vi "Main Tclk.vi"() -> ()   [LabVIEW 2018] (continued)
        n4080 = Select(t=u32[] [16448250, 16711422, 16645629, 16579836, 16514043, 16448250, 16382457, 16316664, 16250871, 16185078, 16119285, 16053492, 15987699, 15921906, 15856113, 15790320, 15724527, 15658734, 15592941, 15527148, 15461355, 15395562, 15329769, 15263976, 15198183, 15132390, 15066597, 15000804, 14935011, 14869218, 14803425, 14737632, 14671839, 14606046, 14540253, 14474460, 14408667, 14342874, 14277081, 14211288, 14145495, 14079702, 14013909, 13948116, 13882323, 13816530, 13750737, 13684944, 13619151, 13553358, 13487565, 13421772, 13355979, 13290186, 13224393, 13158600, 13092807, 13027014, 12961221, 12895428, 12829635, 12763842, 12698049, 12632256, 12566463, 12500670, 12434877, 12369084, 12303291, 12237498, 12171705, 12105912, 12040119, 11974326, 11908533, 11842740, 11776947, 11711154, 11645361, 11579568, 11513775, 11447982, 11382189, 11316396, 11250603, 11184810, 11119017, 11053224, 10987431, 10921638, 10855845, 10790052, 10724259, 10658466, 10592673, 10526880, 10461087, 10395294, 10329501, 10263708, 10197915, 10132122, 10066329, 10000536, 9934743, 9868950, 9803157, 9737364, 9671571, 9605778, 9539985, 9474192, 9408399, 9342606, 9276813, 9211020, 9145227, 9079434, 9013641, 8947848, 8882055, 8816262, 8750469, 8684676, 8618883, 8553090, 8487297, 8421504, 8355711, 8289918, 8224125, 8158332, 8092539, 8026746, 7960953, 7895160, 7829367, 7763574, 7697781, 7631988, 7566195, 7500402, 7434609, 7368816, 7303023, 7237230, 7171437, 7105644, 7039851, 6974058, 6908265, 6842472, 6776679, 6710886, 6645093, 6579300, 6513507, 6447714, 6381921, 6316128, 6250335, 6184542, 6118749, 6052956, 5987163, 5921370, 5855577, 5789784, 5723991, 5658198, 5592405, 5526612, 5460819, 5395026, 5329233, 5263440, 5197647, 5131854, 5066061, 5000268, 4934475, 4868682, 4802889, 4737096, 4671303, 4605510, 4539717, 4473924, 4408131, 4342338, 4276545, 4210752, 4144959, 4079166, 4013373, 3947580, 3881787, 3815994, 3750201, 3684408, 3618615, 3552822, 3487029, 3421236, 3355443, 3289650, 3223857, 3158064, 3092271, 3026478, 2960685, 2894892, 2829099, 2763306, 2697513, 2631720, 2565927, 2500134, 2434341, 2368548, 2302755, 2236962, 2171169, 2105376, 2039583, 1973790, 1907997, 1842204, 1776411, 1710618, 1644825, 1579032, 1513239, 1447446, 1381653, 1315860, 1250067, 1184274, 1118481, 1052688, 986895, 921102, 855309, 789516, 723723, 657930, 592137, 526344, 460551, 394758, 328965, 263172, 197379, 131586, 65793, 16777222] ("256 gray scale inverse"), s=w2804, f=u32[] [16777222, 65793, 131586, 197379, 263172, 328965, 394758, 460551, 526344, 592137, 657930, 723723, 789516, 855309, 921102, 986895, 1052688, 1118481, 1184274, 1250067, 1315860, 1381653, 1447446, 1513239, 1579032, 1644825, 1710618, 1776411, 1842204, 1907997, 1973790, 2039583, 2105376, 2171169, 2236962, 2302755, 2368548, 2434341, 2500134, 2565927, 2631720, 2697513, 2763306, 2829099, 2894892, 2960685, 3026478, 3092271, 3158064, 3223857, 3289650, 3355443, 3421236, 3487029, 3552822, 3618615, 3684408, 3750201, 3815994, 3881787, 3947580, 4013373, 4079166, 4144959, 4210752, 4276545, 4342338, 4408131, 4473924, 4539717, 4605510, 4671303, 4737096, 4802889, 4868682, 4934475, 5000268, 5066061, 5131854, 5197647, 5263440, 5329233, 5395026, 5460819, 5526612, 5592405, 5658198, 5723991, 5789784, 5855577, 5921370, 5987163, 6052956, 6118749, 6184542, 6250335, 6316128, 6381921, 6447714, 6513507, 6579300, 6645093, 6710886, 6776679, 6842472, 6908265, 6974058, 7039851, 7105644, 7171437, 7237230, 7303023, 7368816, 7434609, 7500402, 7566195, 7631988, 7697781, 7763574, 7829367, 7895160, 7960953, 8026746, 8092539, 8158332, 8224125, 8289918, 8355711, 8421504, 8487297, 8553090, 8618883, 8684676, 8750469, 8816262, 8882055, 8947848, 9013641, 9079434, 9145227, 9211020, 9276813, 9342606, 9408399, 9474192, 9539985, 9605778, 9671571, 9737364, 9803157, 9868950, 9934743, 10000536, 10066329, 10132122, 10197915, 10263708, 10329501, 10395294, 10461087, 10526880, 10592673, 10658466, 10724259, 10790052, 10855845, 10921638, 10987431, 11053224, 11119017, 11184810, 11250603, 11316396, 11382189, 11447982, 11513775, 11579568, 11645361, 11711154, 11776947, 11842740, 11908533, 11974326, 12040119, 12105912, 12171705, 12237498, 12303291, 12369084, 12434877, 12500670, 12566463, 12632256, 12698049, 12763842, 12829635, 12895428, 12961221, 13027014, 13092807, 13158600, 13224393, 13290186, 13355979, 13421772, 13487565, 13553358, 13619151, 13684944, 13750737, 13816530, 13882323, 13948116, 14013909, 14079702, 14145495, 14211288, 14277081, 14342874, 14408667, 14474460, 14540253, 14606046, 14671839, 14737632, 14803425, 14869218, 14935011, 15000804, 15066597, 15132390, 15198183, 15263976, 15329769, 15395562, 15461355, 15527148, 15592941, 15658734, 15724527, 15790320, 15856113, 15921906, 15987699, 16053492, 16119285, 16185078, 16250871, 16316664, 16382457, 16448250, 16514043, 16579836, 16645629, 16711422, 16448250] ("256 gray scale")) -> (s? t:f=w2805:u32[])
        n4081 = property on="DetB e- Scaling" class="DigNum (strict)"("Visible"=w2652) -> ()  [unwired: 2 in, 2 out]
        n4082 = property on="Detector B" class="IntGraph (strict)"("Color Table"=w2805, "Caption.Text"=w2840) -> ()  [unwired: 2 in, 2 out]
        n4083 = property on="Det A" class="IntGraph (strict)"("Color Table"=w2806) -> ()  [unwired: 2 in, 2 out]
        n4084 = property on="Align failed array" class="Arr (strict)"("Index Values"=w2701) -> ()  [unwired: 2 in, 2 out]
        n4085 = property on="WD (mm)" class="Arr (strict)"("Index Values"=w2701) -> ()  [unwired: 2 in, 2 out]
        n4086 = property on="X stig" class="Arr (strict)"("Index Values"=w2701) -> ()  [unwired: 2 in, 2 out]
        n4087 = property on="Y stig" class="Arr (strict)"("Index Values"=w2701) -> ()  [unwired: 2 in, 2 out]
        n4088 = property on="X aln" class="Arr (strict)"("Index Values"=w2701) -> ()  [unwired: 2 in, 2 out]
        n4089 = property on="Y aln" class="Arr (strict)"("Index Values"=w2701) -> ()  [unwired: 2 in, 2 out]
        n4090 = property on="Det B" class="IntGraph (strict)"("Color Table"=w2805) -> ()  [unwired: 2 in, 2 out]
        n4091 = property on="Detector A Low Mag" class="IntGraph (strict)"("Color Table"=w2806) -> ()  [unwired: 2 in, 2 out]
        n4092 = local read "FIB"() -> (w2654:bool)
        n4093 = local read "Mill"() -> (w2653:bool)
        n4094 = property on="Detector B Low Mag" class="IntGraph (strict)"("Color Table"=w2805) -> ()  [unwired: 2 in, 2 out]
        n4095 = Or(x=w2654, y=w2653) -> (x .or. y?=w2655:bool)
        n4096 = shared-variable ".\\Zeiss Library.lvlib\\Milling Z Voltage RT"() -> (w2733:sgl)  [unwired: 1 in, 1 out]
        "Milling Z realtime (V)" <- w2733
        n4097 = case shown="True" w2655 {
          tunnel: w2733 -> [_ w2953]
          frame False {
          }
          frame True {
            n4098 = control-ref of="FIB Image"() -> (w2957:refnum<vi>)
            n4099 = local read "FIB Scan Parameters"() -> (w2955:T32)
            n4100 = local read "FIB Options"() -> (w2954:T33)
            n4101 = local read "Milling para"() -> (w2956:T35)
            n4102 = call "FIB image draw milling.vi"("Milling Z Voltage"=w2953, "Milling para"=w2956, "FIB Options"=w2954, "FIB Scan Parameters"=w2955, "Image reference"=w2957) -> ()  [unwired: 5 in, 2 out]
          }
        }
        n4103 = property on="Det A LM" class="IntGraph (strict)"("Color Table"=w2806) -> ()  [unwired: 2 in, 2 out]
        n4104 = property on="Det B LM" class="IntGraph (strict)"("Color Table"=w2805) -> ()  [unwired: 2 in, 2 out]
      }
      n4105 = Open VI Reference(vi path=w709) -> (vi reference=w714:refnum<vi>, error out=w708:errorcluster)  [unwired: 1 in, 4 out]
      n4106 = register-events(error in=w708, refnum<vi> refnum) -> (reference out=w711:refnum<event-registration>)  [unwired: 1 in, 1 out]
      n4107 = local read "Trapezoidal"() -> (w706:cluster{"X":i16, "Y":i16}[])
      n4108 = while {
        stop <- w718 stop-if-true
        n4109 = Wait Until Next ms Multiple(millisecond multiple=u32 100) -> ()  [unwired: 1 out]
        n4110 = case shown="True" "Scan x1" {
          frame False {
          }
          frame True {
            n4111 = Two Button Dialog(message="Single SEM Scan?") -> (T button?=w719:bool)  [unwired: 2 in]
            n4112 = case shown="True" w719 {
              frame False {
                n4113 = local write "Scan x1"(FALSE ("Scan")) -> ()
              }
              frame True {
                n4114 = stacked-sequence {
                  frame #0 {
                    n4115 = local read "SEM Scan Parameters"() -> (w727:T26)
                    n4116 = Unbundle By Name(w727) -> ("WD (mm)"=w728:sgl[][], "X stig"=w731:sgl[][], "Y stig"=w734:sgl[][], "X aln"=w735:sgl[][], "Y aln"=w737:sgl[][], "dX (um)"=w739:sgl[], "dY (um)"=w742:sgl[], "Y tiles"=w724:u8, "X tiles"=w723:u8)
                    n4117 = local read "WD Stig Aln tile offsets"() -> (w725:T3)
                    n4118 = Array Size(array=w728) -> (size(s)=w729:i32[])
                    n4119 = Array Size(array=w731) -> (size(s)=w730:i32[])
                    n4120 = Array Size(array=w734) -> (size(s)=w733:i32[])
                    n4121 = Array Size(array=w735) -> (size(s)=w732:i32[])
                    n4122 = Array Size(array=w737) -> (size(s)=w736:i32[])
                    n4123 = Array Size(array=w739) -> (size(s)=w740:i32)
                    n4124 = Array Size(array=w742) -> (size(s)=w741:i32)
                    n4125 = Build Array(w724, w723) -> (w738:u8[])
                    n4126 = Equal?(x=w729, y=w738) -> (x = y?=w743:bool[])
                    n4127 = Equal?(x=w730, y=w738) -> (x = y?=w744:bool[])
                    n4128 = Equal?(x=w733, y=w738) -> (x = y?=w746:bool[])
                    n4129 = Equal?(x=w732, y=w738) -> (x = y?=w747:bool[])
                    n4130 = Equal?(x=w736, y=w738) -> (x = y?=w748:bool[])
                    n4131 = Equal?(x=w740, y=w724) -> (x = y?=w749:bool)
                    n4132 = Equal?(x=w741, y=w723) -> (x = y?=w750:bool)
                    n4133 = Build Array (concatenate)(w743, w744, w746, w747, w748, w749, w750) -> (w745:bool[])
                    n4134 = And Array Elements(Boolean array=w745) -> (logical AND=w722:bool)
                    n4135 = case shown="True" w722 {
                      tunnel: [w751 w779] -> w726
                      tunnel: w727 -> [w753 w773]
                      tunnel: w725 -> [w752 w760]
                      frame False {
                        w755 = sgl 0.0 ("element")
                        n4136 = Unbundle By Name(w753) -> ("Y tiles"=w757:u8, "X tiles"=w759:u8)
                        n4137 = Initialize Array(w755, w757, w759) -> (w758:sgl[][])
                        n4138 = Initialize Array(w755, w757) -> (w756:sgl[])
                        n4139 = Initialize Array(w755, w759) -> (w754:sgl[])
                        n4140 = Bundle By Name(cluster=w752, "dWD"=w758, "dX stig"=w758, "dY stig"=w758, "dX aln"=w758, "dY aln"=w758, "dX (um)"=w756, "dY (um)"=w754) -> (w751:T3)
                      }
                      frame True {
                        n4141 = Unbundle By Name(w773) -> ("WD (mm)"=w769:sgl[][], "X stig"=w767:sgl[][], "Y stig"=w764:sgl[][], "X aln"=w763:sgl[][], "Y aln"=w761:sgl[][], "dX (um)"=w780:sgl[], "dY (um)"=w785:sgl[], "Y tiles"=w772:u8, "X tiles"=w771:u8)
                        n4142 = expression code="(x-1)/2"(w772) -> (w783:u8)
                        n4143 = expression code="(x-1)/2"(w771) -> (w786:u8)
                        n4144 = Index Array(array=w769, index (row)=w783, index (col)=w786) -> (element=w770:sgl)
                        n4145 = Index Array(array=w767, index (row)=w783, index (col)=w786) -> (element=w768:sgl)
                        n4146 = Index Array(array=w764, index (row)=w783, index (col)=w786) -> (element=w765:sgl)
                        n4147 = Index Array(array=w763, index (row)=w783, index (col)=w786) -> (element=w766:sgl)
                        n4148 = Index Array(array=w761, index (row)=w783, index (col)=w786) -> (element=w762:sgl)
                        n4149 = Index Array(array=w780, index=w783) -> (element=w781:sgl)
                        n4150 = Index Array(array=w785, index=w786) -> (element=w784:sgl)
                        n4151 = Subtract(x=w769, y=w770) -> (x-y=w774:sgl[][])
                        n4152 = Subtract(x=w767, y=w768) -> (x-y=w775:sgl[][])
                        n4153 = Subtract(x=w764, y=w765) -> (x-y=w776:sgl[][])
                        n4154 = Subtract(x=w763, y=w766) -> (x-y=w777:sgl[][])
                        n4155 = Subtract(x=w761, y=w762) -> (x-y=w778:sgl[][])
                        n4156 = Subtract(x=w780, y=w781) -> (x-y=w782:sgl[])
                        n4157 = Subtract(x=w785, y=w784) -> (x-y=w787:sgl[])
                        n4158 = Bundle By Name(cluster=w760, "dWD"=w774, "dX stig"=w775, "dY stig"=w776, "dX aln"=w777, "dY aln"=w778, "dX (um)"=w782, "dY (um)"=w787) -> (w779:T3)
                      }
                    }
                    n4159 = local write "WD Stig Aln tile offsets"(w726) -> ()
                  }
                  frame #1 {
                    n4160 = local read "SEM Scan Parameters"() -> (w793:T26)
                    n4161 = Unbundle By Name(w793) -> ("X tiles"=w789:u8, "Y tiles"=w790:u8)
                    n4162 = Multiply(x=w789, y=w790) -> (x*y=w791:u8)
                    n4163 = Greater?(x=w791, y=u8 1) -> (0:w792:bool)
                    n4164 = case shown="True" w792 {
                      frame False {
                      }
                      frame True {
                        n4165 = local read "Api"() -> (w811:refnum<k7>)
                        n4166 = call "SmartSEM Remote API get float.vi"("lpszParam"="AP_WD", "ActiveX Container"=w811) -> ("error out"=w822:errorcluster, "vValue"=w809:sgl)  [unwired: 7 in, 1 out]
                        n4167 = call "SmartSEM Remote API get float.vi"("error in"=w822, "lpszParam"="AP_STIG_X", "ActiveX Container"=w811) -> ("error out"=w823:errorcluster, "vValue"=w816:sgl, "reference out"=w813:refnum<k7>)  [unwired: 6 in]
                        n4168 = local read "WD Stig Aln tile offsets"() -> (w806:T3)
                        n4169 = expression code="x*1000"(w809) -> (w807:sgl)
                        n4170 = Unbundle By Name(w806) -> ("dWD"=w805:sgl[][], "dX stig"=w804:sgl[][], "dY stig"=w803:sgl[][], "dX aln"=w802:sgl[][], "dY aln"=w801:sgl[][])
                        n4171 = call "SmartSEM Remote API get float.vi"("error in"=w823, "lpszParam"="AP_APERTURE_ALIGN_X", "ActiveX Container"=w813) -> ("error out"=w824:errorcluster, "vValue"=w815:sgl)  [unwired: 6 in, 1 out]
                        n4172 = call "SmartSEM Remote API get float.vi"("error in"=w824, "lpszParam"="AP_STIG_Y", "ActiveX Container"=w811) -> ("error out"=w818:errorcluster, "vValue"=w821:sgl, "reference out"=w817:refnum<k7>)  [unwired: 6 in]
                        n4173 = call "SmartSEM Remote API get float.vi"("error in"=w818, "lpszParam"="AP_APERTURE_ALIGN_Y", "ActiveX Container"=w817) -> ("vValue"=w820:sgl)  [unwired: 6 in, 2 out]
                        n4174 = local read "SEM Scan Parameters"() -> (w799:T26)
                        n4175 = Add(x=w805, y=w807) -> (x+y=w798:sgl[][])
                        n4176 = Add(x=w804, y=w816) -> (x+y=w797:sgl[][])
                        n4177 = Add(x=w803, y=w821) -> (x+y=w796:sgl[][])
                        n4178 = Add(x=w802, y=w815) -> (x+y=w795:sgl[][])
                        n4179 = Add(x=w801, y=w820) -> (x+y=w794:sgl[][])
                        n4180 = Bundle By Name(cluster=w799, "WD (mm)"=w798, "X stig"=w797, "Y stig"=w796, "X aln"=w795, "Y aln"=w794) -> (w800:T26)
                        n4181 = local write "SEM Scan Parameters"(w800) -> ()
                      }
                    }
                  }
                  frame #2 {
                    n4182 = local read "SEM HW Config"() -> (w850:T9)
                    n4183 = local read "Detector Information"() -> (w849:T8)
                    n4184 = local read "SEM Scan Parameters"() -> (w837:T26)
                    n4185 = local read "SEM Options"() -> (w847:T27)
                    n4186 = local read "Focus Index Options"() -> (w846:T28)
                    n4187 = local read "File Information"() -> (w845:T31)
                    n4188 = local read "Milling para"() -> (w844:T35)
                    n4189 = Bundle By Name(cluster="Tiled scan inputs", "HW Config"=w850, "Det Info"=w849, "SEM Scan Parameters"=w837, "SEM Options"=w847, "Focus Index Options"=w846, "File Information"=w845, "Milling para"=w844, "Additional Info"=cluster{"Restart flag":u8, "Stage move flag":u8} {"Restart flag"=100, "Stage move flag"=100}) -> (w839:T6)
                    n4190 = Unbundle By Name(w837) -> ("X tiles"=w836:u8, "Y tiles"=w835:u8)
                    n4191 = Multiply(x=w836, y=w835) -> (x*y=w834:u8)
                    n4192 = Greater?(x=w834, y=u8 1) -> (0:w833:bool)
                    n4193 = local read "WatchDog Mode"() -> (w852:u16)
                    n4194 = case shown="True" w833 {
                      tunnel: w839 -> [w862 w865]
                      tunnel: [w862 w863] -> w838
                      frame False {
                      }
                      frame True {
                        w864 = TRUE ("SEM Options.Set WD")
                        n4195 = Bundle By Name(cluster=w865, "SEM Options.Set WD"=w864, "SEM Options.Set stig"=w864, "SEM Options.Set aln"=w864) -> (w863:T6)
                      }
                    }
                    n4196 = local read "Api"() -> (w851:refnum<k7>)
                    n4197 = call "2D scan tiled.vi"("WatchDog Mode"=w852, "Tiled scan inputs"=w838, "ActiveX Container"=w851) -> ("Image Focus Index Tiled"=w840:T53, "Image Focus Index Array Tiled"=w841:T54, "Single scan outputs"=w860:T55, "8-bit over scale"=w857:bool[])  [unwired: 3 in, 2 out]
                    n4198 = local read "FI Detector"() -> (w843:u16)
                    n4199 = Index Array(array=w857, index #1=0 ("index"), index #2=1 ("index")) -> (element #1=→"Det A over scale":bool, element #2=→"Det B over scale":bool)
                    n4200 = case shown="1" w843 {
                      tunnel: w840 -> [w869 w873 w877 w881]
                      tunnel: [w868 w870 w876 w880] -> w827
                      tunnel: w841 -> [w866 w872 w875 w879]
                      tunnel: [w867 w871 w874 w878] -> w842
                      frame 0, Default {
                        n4201 = Unbundle By Name(w869) -> ("A Img Focus Index"=w868:sgl[][])
                        n4202 = Unbundle By Name(w866) -> ("A Img Focus Index array"=w867:sgl[][][][])
                      }
                      frame 1 {
                        n4203 = Unbundle By Name(w873) -> ("B Img Focus Index"=w870:sgl[][])
                        n4204 = Unbundle By Name(w872) -> ("B Img Focus Index array"=w871:sgl[][][][])
                      }
                      frame 2 {
                        n4205 = Unbundle By Name(w877) -> ("C Img Focus Index"=w876:sgl[][])
                        n4206 = Unbundle By Name(w875) -> ("C Img Focus Index array"=w874:sgl[][][][])
                      }
                      frame 3 {
                        n4207 = Unbundle By Name(w881) -> ("D Img Focus Index"=w880:sgl[][])
                        n4208 = Unbundle By Name(w879) -> ("D Img Focus Index array"=w878:sgl[][][][])
                      }
                    }
                    n4209 = Unbundle By Name(w860) -> ("SEM Parameters"=→"SEM Parameters":T13, "Image Focus Index"=→"Image Focus Index":T14)
                    n4210 = Array Size(array=w827) -> (size(s)=w828:i32[])
                    n4211 = local write "Focus Index tiled"(w827) -> ()
                    n4212 = local write "Focus Index array tiled"(w842) -> ()
                    n4213 = local write "FRC resolution"(sgl 0.0 ("FRC resolution")) -> ()
                    n4214 = Multiply Array Elements(1:w828) -> (0:w829:i32)
                    n4215 = Reshape Array(w827, w829) -> (w830:sgl[])
                    n4216 = call-poly <vilib>:"Mean.vi"("X"=w830) -> ("mean"=w831:dbl)  [unwired: 1 out]
                    n4217 = local write "Focus Index"(w831) -> ()
                    "Status message" <- "SEM scanning" ("Status message")
                  }
                  frame #3 {
                    n4218 = local write "Scan x1"(FALSE ("Scan")) -> ()
                    n4219 = local write "Status message"("Single scan finished." ("Status message")) -> ()
                  }
                }
              }
            }
          }
        }
        n4220 = local read "Stop"() -> (w718:bool)
      }
      n4221 = while {
        tunnel: w711 -> [w3157]
        tunnel: [w3156] -> w712
        tunnel: [w3154] -> w713
        tunnel: w714 -> [w3155]
        shift-right: [w3149] -> _
        shift-left: w706 -> [w3148]
        stop <- w3153 stop-if-true
        n4222 = Wait Until Next ms Multiple(millisecond multiple=u32 1) -> ()  [unwired: 1 out]
        n4223 = event shown="[24] \"Mill\": Value Change" {
          selector: w3157 -> [_ _ _ _ _ _ _ _ _ _ _ _ _ _ _ _ _ _ _ _ _ _ _ _ _ _ _ _ _ _ _ _ w3973 _ w4176 _ _ _ _ _ _ _ _ _ _ _ _ _ _ _ _ _ _ _ _ _ _ _ _ _ _ _ _ _ _ _ _ _ _ _ _ _ _ _ _ _ _ _ _ _ _ _ _ _ _ _ _ _ _ _ _ _ _ _]
          dyn-events: [_ _ _ _ _ _ _ _ _ _ _ _ _ _ _ _ _ _ _ _ _ _ _ _ _ _ _ _ _ _ _ _ w3972 _ w4175 _ _ _ _ _ _ _ _ _ _ _ _ _ _ _ _ _ _ _ _ _ _ _ _ _ _ _ _ _ _ _ _ _ _ _ _ _ _ _ _ _ _ _ _ _ _ _ _ _ _ _ _ _ _ _ _ _ _ _] -> w3156
          timeout: _ -> [_ _ _ _ _ _ _ _ _ _ _ _ _ _ _ _ _ _ _ _ _ _ _ _ _ _ _ _ _ _ _ _ _ _ _ _ _ _ _ _ _ _ _ _ _ _ _ _ _ _ _ _ _ _ _ _ _ _ _ _ _ _ _ _ _ _ _ _ _ _ _ _ _ _ _ _ _ _ _ _ _ _ _ _ _ _ _ _ _ _ _ _ _ _]
          tunnel: [_ _ _ _ _ _ _ _ _ _ _ _ _ _ _ _ _ _ _ _ _ _ _ _ _ _ _ _ _ _ _ _ w3971 _ w4174 _ _ _ _ _ _ _ _ _ _ _ _ _ _ _ _ _ _ _ _ _ _ _ _ _ _ _ _ _ _ _ _ _ _ _ _ _ _ _ _ _ _ _ _ _ _ _ _ _ _ _ _ _ _ _ _ _ _ _] -> w3154
          tunnel: w3155 -> [_ _ _ _ _ _ _ _ _ _ _ _ _ _ _ _ _ _ _ _ _ _ _ _ _ _ _ _ _ _ _ _ w3969 _ _ _ _ _ _ _ _ _ _ _ _ _ _ _ _ _ _ _ _ _ _ _ _ _ _ _ _ _ _ _ _ _ _ _ _ _ _ _ _ _ _ _ _ _ _ _ _ _ _ _ _ _ _ _ _ _ _ _ _ _]
          tunnel: [_ _ _ _ _ _ _ _ _ _ _ w3510 _ _ _ _ _ _ _ _ _ _ _ _ _ _ _ _ _ _ _ _ _ _ _ _ _ _ _ _ _ _ _ _ _ _ _ _ _ _ _ _ _ _ _ _ _ _ _ _ _ _ _ _ _ _ _ _ _ _ _ _ _ _ _ _ _ _ _ _ _ _ _ _ _ _ _ _ _ _ _ _ _ _] -> w3151
          tunnel: [_ _ _ _ _ _ _ _ _ _ _ _ _ _ _ _ _ _ _ _ _ _ _ _ _ _ _ _ _ _ _ _ w3965 w3984 w4140 _ _ _ w4309 _ _ _ _ _ _ _ _ w4788 _ _ _ _ _ _ _ _ _ _ _ _ _ _ _ _ _ _ _ _ _ _ _ _ _ _ _ _ _ _ _ _ _ _ _ _ _ _ _ _ _ _ _ _ _ _] -> w3149
          tunnel: w3148 -> [_ _ _ _ _ _ _ _ _ _ _ _ _ _ _ _ _ _ _ _ _ _ _ _ _ _ _ _ _ _ _ _ w3965 w3983 w4140 _ _ _ _ _ _ _ _ _ _ _ _ w4787 _ _ _ _ _ _ _ _ _ _ _ _ _ _ _ _ _ _ _ _ _ _ _ _ _ _ _ _ _ _ _ _ _ _ _ _ _ _ _ _ _ _ _ _ _ _]
          event Timeout {
            n4224 = event-data() -> ()  [unwired: 3 out]
          }
          event Key Down? {
            # "Ignore Ctrl-W, Alt-F4"
            n4225 = event-data() -> ("Char"=w3169:i16, "VKey"=w3166:T48, "PlatMods"=w3164:T77)  [unwired: 7 out]
            n4226 = Unbundle By Name(w3164) -> ("Ctrl"=w3163:bool, "Alt"=w3161:bool)
            n4227 = Equal?(x=w3169, y=i16 119) -> (x = y?=w3167:bool)
            n4228 = Equal?(x=w3166, y=eventvkey."F4" ("VKey")) -> (x = y?=w3162:bool)
            n4229 = And(x=w3167, y=w3163) -> (x .and. y?=w3160:bool)
            n4230 = And(x=w3161, y=w3162) -> (x .and. y?=w3159:bool)
            n4231 = Compound Arithmetic op=OR(w3160, w3159) -> (w3158:bool)
            n4232 = event-data("Discard?"=w3158) -> ()  [unwired: 6 in, 1 out]
          }
          event "Hardware Configuration", "SEM Options", "Mid Mag SEM", "SEM Scan Parameters.Scan rate (Hz)", "SEM Scan Parameters.Oversampling", "SEM Scan Parameters.Oversampling auto", "SEM Scan Parameters.X size (um)", "SEM Scan Parameters.X size (V)", "SEM Scan Parameters.X size auto", "SEM Scan Parameters.Y size (um)", "SEM Scan Parameters.X center (um)", "SEM Scan Parameters.Y center (um)": Value Change {
            n4233 = event-data() -> ()  [unwired: 6 out]
            n4234 = local read "Hardware Configuration"() -> (w3178:T25)
            n4235 = local read "SEM Scan Parameters"() -> (w3194:T26)
            n4236 = local read "SEM Options"() -> (w3177:T27)
            n4237 = local read "SEM Status"() -> (w3176:T12)
            n4238 = local read "X full scale (V)"() -> (w3175:sgl)
            n4239 = local read "Mid Mag SEM"() -> (w3179:T29)
            n4240 = local read "SEM Mid Mag Scan Parameters"() -> (w3180:T5)
            n4241 = Unbundle By Name(w3179) -> ("X size (um)"=w3183:sgl, "Y size (um)"=w3184:sgl, "X center (um)"=w3185:dbl, "Y center (um)"=w3186:dbl, "Mid mag scan rate (Hz)"=w3181:u32, "Pixel size (nm)"=w3182:sgl)
            n4242 = call "SEM Scan Parameter Coerce.vi"("X full scale (V)"=w3175, "AI upper limit"=50000000.0, "SEM Status"=w3176, "SEM Options"=w3177, "SEM Scan Parameters"=w3194, "Hardware Configuration"=w3178) -> ("Coerced SEM Scan Parameters"=w3174:T5, "SEM FOV"=→"SEM FOV":dbl, "Detector number"=→"Detector number":i16)  [unwired: 3 in]
            n4243 = Bundle By Name(cluster=w3180, "X size (um)"=w3183, "Y size (um)"=w3184, "X center (um)"=w3185, "Y center (um)"=w3186, "Scan rate (Hz)"=w3181, "Pixel size (nm)"=w3182, "X size auto"=TRUE) -> (w3187:T5)
            n4244 = call "SEM Scan Parameter Coerce.vi"("X full scale (V)"=w3175, "SEM Status"=w3176, "SEM Options"=w3177, "SEM Scan Parameters"=w3187, "Hardware Configuration"=w3178) -> ("Coerced SEM Scan Parameters"=w3173:T5)  [unwired: 4 in, 2 out]
            n4245 = Unbundle By Name(w3173) -> ("X size (um)"=w3188:sgl, "Y size (um)"=w3189:sgl, "X center (um)"=w3190:dbl, "Y center (um)"=w3191:dbl, "Scan rate (Hz)"=w3192:u32, "Pixel size (nm)"=w3193:sgl)
            n4246 = Bundle By Name(cluster=w3179, "X size (um)"=w3188, "Y size (um)"=w3189, "X center (um)"=w3190, "Y center (um)"=w3191, "Mid mag scan rate (Hz)"=w3192, "Pixel size (nm)"=w3193) -> (w3172:T29)
            n4247 = local write "SEM Scan Parameters"(w3174) -> ()
            n4248 = local write "SEM Mid Mag Scan Parameters"(w3173) -> ()
            n4249 = local write "Mid Mag SEM"(w3172) -> ()
          }
          event "Scan x1": Value Change {
            n4250 = event-data() -> ()  [unwired: 6 out]
          }
          event "3D FIB-SEM": Value Change {
            n4251 = event-data() -> ("NewVal"=w3197:bool)  [unwired: 5 out]
            n4252 = case shown="False" w3197 {
              frame False {
                n4253 = Two Button Dialog(message="Stop 3D FIB-SEM?") -> (T button?=w3198:bool)  [unwired: 2 in]
                n4254 = local write "Mill Stop"(w3198) -> ()
                n4255 = case shown="True" w3198 {
                  frame False {
                    n4256 = local write "3D FIB-SEM"(TRUE ("3D FIB-SEM")) -> ()
                  }
                  frame True {
                    n4257 = stacked-sequence {
                      frame #0 {
                        n4258 = shared-variable "My Computer\\Zeiss Library.lvlib\\Milling Stop"(TRUE ("Milling Stop")) -> ()  [unwired: 1 in, 1 out]
                        n4259 = Wait (ms)(milliseconds to wait=u32 1000) -> ()  [unwired: 1 out]
                        n4260 = local write "Status message"("3D FIB-SEM stopped" ("Status message")) -> ()
                        n4261 = local read "WatchDog Mode"() -> (w3201:u16)
                        n4262 = call "FM Gen Pulse for FIB-SEM.vi"("WatchDog Mode"=w3201, "State Value"=i16 7) -> ()  [unwired: 7 in, 3 out]
                      }
                      frame #1 {
                        w3206 = FALSE ("3D FIB-SEM")
                        n4263 = local read "Last FIB recipe"() -> (w3216:path)
                        n4264 = local read "Email recipents file"() -> (w3210:path)
                        n4265 = local read "FIB Image"() -> (w3221:i16[][])
                        n4266 = Array Size(array=w3221) -> (size(s)=w3220:i32[])
                        n4267 = local write "Pause for reheat"(w3206) -> ()
                        n4268 = local write "3D FIB-SEM"(w3206) -> ()
                        n4269 = local write "FIB"(w3206) -> ()
                        n4270 = Add Array Elements(numeric array=w3220) -> (sum=w3219:i32)
                        n4271 = Not Equal To 0?(x=w3219) -> (x != 0?=w3218:bool)
                        n4272 = Open/Create/Replace File(file path (use dialog)=w3216) -> (error out=w3214:errorcluster)  [unwired: 5 in, 2 out]
                        n4273 = case shown="True" w3218 {
                          tunnel: w3221 -> [_ w3247]
                          frame False {
                          }
                          frame True {
                            n4274 = local read "Last FIB image"() -> (w3250:path)
                            n4275 = call "16bit Image Normalization.vi"("Transpose"=FALSE, "Input image"=w3247) -> ("Normalized image"=w3246:u8[][])  [unwired: 5 in, 4 out]
                            n4276 = call <vilib>:"Flatten Pixmap.vi"("colors"=u32[] [16777222, 65793, 131586, 197379, 263172, 328965, 394758, 460551, 526344, 592137, 657930, 723723, 789516, 855309, 921102, 986895, 1052688, 1118481, 1184274, 1250067, 1315860, 1381653, 1447446, 1513239, 1579032, 1644825, 1710618, 1776411, 1842204, 1907997, 1973790, 2039583, 2105376, 2171169, 2236962, 2302755, 2368548, 2434341, 2500134, 2565927, 2631720, 2697513, 2763306, 2829099, 2894892, 2960685, 3026478, 3092271, 3158064, 3223857, 3289650, 3355443, 3421236, 3487029, 3552822, 3618615, 3684408, 3750201, 3815994, 3881787, 3947580, 4013373, 4079166, 4144959, 4210752, 4276545, 4342338, 4408131, 4473924, 4539717, 4605510, 4671303, 4737096, 4802889, 4868682, 4934475, 5000268, 5066061, 5131854, 5197647, 5263440, 5329233, 5395026, 5460819, 5526612, 5592405, 5658198, 5723991, 5789784, 5855577, 5921370, 5987163, 6052956, 6118749, 6184542, 6250335, 6316128, 6381921, 6447714, 6513507, 6579300, 6645093, 6710886, 6776679, 6842472, 6908265, 6974058, 7039851, 7105644, 7171437, 7237230, 7303023, 7368816, 7434609, 7500402, 7566195, 7631988, 7697781, 7763574, 7829367, 7895160, 7960953, 8026746, 8092539, 8158332, 8224125, 8289918, 8355711, 8421504, 8487297, 8553090, 8618883, 8684676, 8750469, 8816262, 8882055, 8947848, 9013641, 9079434, 9145227, 9211020, 9276813, 9342606, 9408399, 9474192, 9539985, 9605778, 9671571, 9737364, 9803157, 9868950, 9934743, 10000536, 10066329, 10132122, 10197915, 10263708, 10329501, 10395294, 10461087, 10526880, 10592673, 10658466, 10724259, 10790052, 10855845, 10921638, 10987431, 11053224, 11119017, 11184810, 11250603, 11316396, 11382189, 11447982, 11513775, 11579568, 11645361, 11711154, 11776947, 11842740, 11908533, 11974326, 12040119, 12105912, 12171705, 12237498, 12303291, 12369084, 12434877, 12500670, 12566463, 12632256, 12698049, 12763842, 12829635, 12895428, 12961221, 13027014, 13092807, 13158600, 13224393, 13290186, 13355979, 13421772, 13487565, 13553358, 13619151, 13684944, 13750737, 13816530, 13882323, 13948116, 14013909, 14079702, 14145495, 14211288, 14277081, 14342874, 14408667, 14474460, 14540253, 14606046, 14671839, 14737632, 14803425, 14869218, 14935011, 15000804, 15066597, 15132390, 15198183, 15263976, 15329769, 15395562, 15461355, 15527148, 15592941, 15658734, 15724527, 15790320, 15856113, 15921906, 15987699, 16053492, 16119285, 16185078, 16250871, 16316664, 16382457, 16448250, 16514043, 16579836, 16645629, 16711422, 16448250] ("256 gray scale"), "8-bit pixmap"=w3246) -> ("image data"=w3249:T52)  [unwired: 4 in, 5 out]
                            n4277 = call <vilib>:"Write PNG File.vi"("image data"=w3249, "path to PNG file"=w3250) -> ()  [unwired: 1 in, 9 out]
                          }
                        }
                        n4278 = File/Directory Info(path=w3210) -> (path out=w3207:path, error out=w3209:errorcluster)  [unwired: 1 in, 5 out]
                        n4279 = Unbundle By Name(w3214) -> ("status"=w3215:bool)
                        n4280 = Unbundle By Name(w3209) -> ("status"=w3208:bool)
                        n4281 = local read "Recipe input"() -> (w3212:T7)
                        n4282 = case shown="False" w3215 {
                          tunnel: w3216 -> [w3244 w3245]
                          tunnel: [w3243 w3245] -> w3213
                          frame False {
                            n4283 = Delete(path (use dialog)=w3244) -> (deleted path=w3243:path)  [unwired: 4 in, 2 out]
                          }
                          frame True {
                          }
                        }
                        n4284 = case shown="False" w3208 {
                          tunnel: w3207 -> [w3230 _]
                          frame False {
                            n4285 = Delete(path (use dialog)=w3230) -> ()  [unwired: 4 in, 3 out]
                          }
                          frame True {
                          }
                        }
                        n4286 = call "Recipe read write.vi"("Write"=TRUE, "Recipe path"=w3213, "Write input"=w3212) -> ()  [unwired: 5 in, 4 out]
                        n4287 = local read "Detector A Low Mag"() -> (w3223:i16[][])
                        n4288 = local read "Detector B Low Mag"() -> (w3222:i16[][])
                        n4289 = Array Size(array=w3223) -> (size(s)=w3224:i32[])
                        n4290 = Array Size(array=w3222) -> (size(s)=w3229:i32[])
                        n4291 = Add Array Elements(numeric array=w3224) -> (sum=w3225:i32)
                        n4292 = Add Array Elements(numeric array=w3229) -> (sum=w3228:i32)
                        n4293 = Not Equal To 0?(x=w3225) -> (x != 0?=w3226:bool)
                        n4294 = Not Equal To 0?(x=w3228) -> (x != 0?=w3227:bool)
                        n4295 = case shown="True" w3226 {
                          tunnel: w3223 -> [_ w3239]
                          frame False {
                          }
                          frame True {
                            n4296 = local read "Last Det A Low Mag"() -> (w3241:path)
                            n4297 = call "16bit Image Normalization.vi"("Transpose"=FALSE, "Input image"=w3239) -> ("Normalized image"=w3238:u8[][])  [unwired: 5 in, 4 out]
                            n4298 = call <vilib>:"Flatten Pixmap.vi"("colors"=u32[] [16777222, 65793, 131586, 197379, 263172, 328965, 394758, 460551, 526344, 592137, 657930, 723723, 789516, 855309, 921102, 986895, 1052688, 1118481, 1184274, 1250067, 1315860, 1381653, 1447446, 1513239, 1579032, 1644825, 1710618, 1776411, 1842204, 1907997, 1973790, 2039583, 2105376, 2171169, 2236962, 2302755, 2368548, 2434341, 2500134, 2565927, 2631720, 2697513, 2763306, 2829099, 2894892, 2960685, 3026478, 3092271, 3158064, 3223857, 3289650, 3355443, 3421236, 3487029, 3552822, 3618615, 3684408, 3750201, 3815994, 3881787, 3947580, 4013373, 4079166, 4144959, 4210752, 4276545, 4342338, 4408131, 4473924, 4539717, 4605510, 4671303, 4737096, 4802889, 4868682, 4934475, 5000268, 5066061, 5131854, 5197647, 5263440, 5329233, 5395026, 5460819, 5526612, 5592405, 5658198, 5723991, 5789784, 5855577, 5921370, 5987163, 6052956, 6118749, 6184542, 6250335, 6316128, 6381921, 6447714, 6513507, 6579300, 6645093, 6710886, 6776679, 6842472, 6908265, 6974058, 7039851, 7105644, 7171437, 7237230, 7303023, 7368816, 7434609, 7500402, 7566195, 7631988, 7697781, 7763574, 7829367, 7895160, 7960953, 8026746, 8092539, 8158332, 8224125, 8289918, 8355711, 8421504, 8487297, 8553090, 8618883, 8684676, 8750469, 8816262, 8882055, 8947848, 9013641, 9079434, 9145227, 9211020, 9276813, 9342606, 9408399, 9474192, 9539985, 9605778, 9671571, 9737364, 9803157, 9868950, 9934743, 10000536, 10066329, 10132122, 10197915, 10263708, 10329501, 10395294, 10461087, 10526880, 10592673, 10658466, 10724259, 10790052, 10855845, 10921638, 10987431, 11053224, 11119017, 11184810, 11250603, 11316396, 11382189, 11447982, 11513775, 11579568, 11645361, 11711154, 11776947, 11842740, 11908533, 11974326, 12040119, 12105912, 12171705, 12237498, 12303291, 12369084, 12434877, 12500670, 12566463, 12632256, 12698049, 12763842, 12829635, 12895428, 12961221, 13027014, 13092807, 13158600, 13224393, 13290186, 13355979, 13421772, 13487565, 13553358, 13619151, 13684944, 13750737, 13816530, 13882323, 13948116, 14013909, 14079702, 14145495, 14211288, 14277081, 14342874, 14408667, 14474460, 14540253, 14606046, 14671839, 14737632, 14803425, 14869218, 14935011, 15000804, 15066597, 15132390, 15198183, 15263976, 15329769, 15395562, 15461355, 15527148, 15592941, 15658734, 15724527, 15790320, 15856113, 15921906, 15987699, 16053492, 16119285, 16185078, 16250871, 16316664, 16382457, 16448250, 16514043, 16579836, 16645629, 16711422, 16448250] ("256 gray scale"), "8-bit pixmap"=w3238) -> ("image data"=w3240:T52)  [unwired: 4 in, 5 out]
                            n4299 = call <vilib>:"Write PNG File.vi"("image data"=w3240, "path to PNG file"=w3241) -> ()  [unwired: 1 in, 9 out]
                          }
                        }
                        n4300 = case shown="True" w3227 {
                          tunnel: w3222 -> [_ w3232]
                          frame False {
                          }
                          frame True {
                            n4301 = local read "Last Det B Low Mag"() -> (w3235:path)
                            n4302 = call "16bit Image Normalization.vi"("Transpose"=FALSE, "Input image"=w3232) -> ("Normalized image"=w3231:u8[][])  [unwired: 5 in, 4 out]
                            n4303 = call <vilib>:"Flatten Pixmap.vi"("colors"=u32[] [16777222, 65793, 131586, 197379, 263172, 328965, 394758, 460551, 526344, 592137, 657930, 723723, 789516, 855309, 921102, 986895, 1052688, 1118481, 1184274, 1250067, 1315860, 1381653, 1447446, 1513239, 1579032, 1644825, 1710618, 1776411, 1842204, 1907997, 1973790, 2039583, 2105376, 2171169, 2236962, 2302755, 2368548, 2434341, 2500134, 2565927, 2631720, 2697513, 2763306, 2829099, 2894892, 2960685, 3026478, 3092271, 3158064, 3223857, 3289650, 3355443, 3421236, 3487029, 3552822, 3618615, 3684408, 3750201, 3815994, 3881787, 3947580, 4013373, 4079166, 4144959, 4210752, 4276545, 4342338, 4408131, 4473924, 4539717, 4605510, 4671303, 4737096, 4802889, 4868682, 4934475, 5000268, 5066061, 5131854, 5197647, 5263440, 5329233, 5395026, 5460819, 5526612, 5592405, 5658198, 5723991, 5789784, 5855577, 5921370, 5987163, 6052956, 6118749, 6184542, 6250335, 6316128, 6381921, 6447714, 6513507, 6579300, 6645093, 6710886, 6776679, 6842472, 6908265, 6974058, 7039851, 7105644, 7171437, 7237230, 7303023, 7368816, 7434609, 7500402, 7566195, 7631988, 7697781, 7763574, 7829367, 7895160, 7960953, 8026746, 8092539, 8158332, 8224125, 8289918, 8355711, 8421504, 8487297, 8553090, 8618883, 8684676, 8750469, 8816262, 8882055, 8947848, 9013641, 9079434, 9145227, 9211020, 9276813, 9342606, 9408399, 9474192, 9539985, 9605778, 9671571, 9737364, 9803157, 9868950, 9934743, 10000536, 10066329, 10132122, 10197915, 10263708, 10329501, 10395294, 10461087, 10526880, 10592673, 10658466, 10724259, 10790052, 10855845, 10921638, 10987431, 11053224, 11119017, 11184810, 11250603, 11316396, 11382189, 11447982, 11513775, 11579568, 11645361, 11711154, 11776947, 11842740, 11908533, 11974326, 12040119, 12105912, 12171705, 12237498, 12303291, 12369084, 12434877, 12500670, 12566463, 12632256, 12698049, 12763842, 12829635, 12895428, 12961221, 13027014, 13092807, 13158600, 13224393, 13290186, 13355979, 13421772, 13487565, 13553358, 13619151, 13684944, 13750737, 13816530, 13882323, 13948116, 14013909, 14079702, 14145495, 14211288, 14277081, 14342874, 14408667, 14474460, 14540253, 14606046, 14671839, 14737632, 14803425, 14869218, 14935011, 15000804, 15066597, 15132390, 15198183, 15263976, 15329769, 15395562, 15461355, 15527148, 15592941, 15658734, 15724527, 15790320, 15856113, 15921906, 15987699, 16053492, 16119285, 16185078, 16250871, 16316664, 16382457, 16448250, 16514043, 16579836, 16645629, 16711422, 16448250] ("256 gray scale"), "8-bit pixmap"=w3231) -> ("image data"=w3234:T52)  [unwired: 4 in, 5 out]
                            n4304 = call <vilib>:"Write PNG File.vi"("image data"=w3234, "path to PNG file"=w3235) -> ()  [unwired: 1 in, 9 out]
                          }
                        }
                        n4305 = property on="Pause for reheat" class="Bool (strict)"("DisabledEnum"=T44."Disabled and Grayed Out" ("Disabled")) -> ()  [unwired: 2 in, 2 out]
                      }
                    }
                  }
                }
              }
              frame True {
                # "Issue the reset pulses and wait 250 mSec to be sure no other\npulses get sent which would over-ride the reset pulse."
                n4306 = local read "Milling para"() -> (w3255:T35)
                n4307 = local read "Machine Type"() -> (w3253:u8)
                n4308 = Unbundle By Name(w3255) -> ("Mill start from Last"=w3254:bool)
                n4309 = case shown="2" w3253 {
                  frame 0, Default {
                  }
                  frame 2 {
                    n4310 = stacked-sequence {
                      frame #0 {
                        n4311 = local read "Api"() -> (w3268:refnum<k7>)
                        n4312 = local read "FIB Milling Probe"() -> (w3266:string)
                        n4313 = call "SmartSEM Remote API set string.vi"("vValue"=w3266, "lpszParam"="DP_FIB_IMAGE_PROBE", "ActiveX Container"=w3268) -> ()  [unwired: 7 in, 2 out]
                      }
                      frame #1 {
                        n4314 = while {
                          i -> [w3273]
                          stop <- w3270 stop-if-true
                          n4315 = local read "Api"() -> (w3277:refnum<k7>)
                          n4316 = local read "FIB Milling Probe"() -> (w3274:string)
                          n4317 = Wait (ms)(milliseconds to wait=u32 500 ("millisecond multiple")) -> ()  [unwired: 1 out]
                          n4318 = Greater?(x=w3273, y=4) -> (0:w3269:bool)
                          n4319 = call "SmartSEM Remote API get string.vi"("lpszParam"="DP_FIB_IMAGE_PROBE", "ActiveX Container"=w3277) -> ("data"=w3275:string)  [unwired: 7 in, 2 out]
                          n4320 = Equal?(x=w3275, y=w3274) -> (x = y?=w3271:bool)
                          n4321 = Or(x=w3271, y=w3269) -> (x .or. y?=w3270:bool)
                        }
                      }
                      frame #2 {
                        n4322 = local read "Api"() -> (w3279:refnum<k7>)
                        n4323 = call "SmartSEM Remote API set float.vi"("vValue"="FIB Milling Objective (V)", "lpszParam"="AP_FIB_OBJECTIVE_POTENTIAL", "ActiveX Container"=w3279) -> ()  [unwired: 7 in, 2 out]
                      }
                    }
                  }
                }
                n4324 = Two Button Dialog(message="Confirm FIB milling probe,\nand start 3D FIB-SEM?") -> (T button?=w3257:bool)  [unwired: 2 in]
                n4325 = And(x=w3257, y=w3254) -> (x .and. y?=w3258:bool)
                n4326 = case shown="False" w3258 {
                  tunnel: w3257 -> [w3282 w3287]
                  tunnel: [w3282 w3287] -> w3256
                  frame False {
                  }
                  frame True {
                    n4327 = Two Button Dialog(message="Are you sure to resume from the last recipe and milling position?") -> (T button?=w3283:bool)  [unwired: 2 in]
                    n4328 = local read "Milling para"() -> (w3284:T35)
                    n4329 = Bundle By Name(cluster=w3284, "Mill start from Last"=w3283) -> (w3285:T35)
                    n4330 = local write "Milling para"(w3285) -> ()
                  }
                }
                n4331 = local read "WatchDog Mode"() -> (w3252:u16)
                n4332 = flat-sequence {
                  tunnel: w3252 -> [w3260]
                  tunnel: w3252 -> [w3263]
                  frame #0 {
                    n4333 = call "FM Gen Pulse for FIB-SEM.vi"("WatchDog Mode"=w3260, "State Value"=i16 0) -> ()  [unwired: 7 in, 3 out]
                  }
                  frame #1 {
                    n4334 = Wait (ms)(milliseconds to wait=u32 2) -> ()  [unwired: 1 out]
                  }
                  frame #2 {
                    n4335 = call "FM Gen Pulse for FIB-SEM.vi"("WatchDog Mode"=w3263, "State Value"=i16 1) -> ()  [unwired: 7 in, 3 out]
                  }
                  frame #3 {
                    n4336 = Wait (ms)(milliseconds to wait=u32 250) -> ()  [unwired: 1 out]
                  }
                }
                n4337 = case shown="True" w3256 {
                  frame False {
                  }
                  frame True {
                    n4338 = local read "Hardware Configuration"() -> (w3291:T25)
                    n4339 = local read "Email Alert Recipients"() -> (w3304:string[])
                    n4340 = local read "Email recipents file"() -> (w3301:path)
                    n4341 = Unbundle By Name(w3291) -> ("Shutter Drive"=w3297:tag)
                    n4342 = local read "Damping"() -> (w3290:bool)
                    n4343 = local write "FIB slice #"(u32 0 ("slice #")) -> ()
                    n4344 = local write "Start FIB HV DataLog"(TRUE ("Start FIB HV DataLog")) -> ()
                    n4345 = local write "Status Tabs"(T11."Status" ("Status Tabs")) -> ()
                    n4346 = Open/Create/Replace File(file path (use dialog)=w3301, operation (0:open)=T49."replace or create") -> (refnum out=w3302:refnum<file>, error out=w3303:errorcluster)  [unwired: 4 in, 1 out]
                    n4347 = call "Shutter Swing V3.vi"("Shutter Drive"=w3297, "Damping"=w3290, "Shutter close"=TRUE) -> ("Shutter close fdbk"=w3296:bool, "Fail #"=w3293:u8, "SEM shutter status"=w3292:string)  [unwired: 2 in, 4 out]
                    n4348 = Write to Text File(file (use dialog)=w3302, text=w3304, error in=w3303) -> (refnum out=w3305:refnum<file>, error out=w3306:errorcluster)  [unwired: 1 in, 1 out]
                    n4349 = Greater Than 0?(x=w3293) -> (x > 0?=w3295:bool)
                    n4350 = local read "WatchDog Mode"() -> (w3288:u16)
                    n4351 = Close File(refnum=w3305, error in=w3306) -> ()  [unwired: 2 out]
                    n4352 = local write "SEM shutter status"(w3292) -> ()
                    n4353 = local write "Fail #"(w3293) -> ()
                    n4354 = local write "SEM shutter failed active"(w3295) -> ()
                    n4355 = local write "SEM Shutter"(w3296) -> ()
                    n4356 = call "FM Gen Pulse for FIB-SEM.vi"("WatchDog Mode"=w3288, "State Value"=i16 6) -> ()  [unwired: 7 in, 3 out]
                  }
                }
                n4357 = local write "3D FIB-SEM"(w3256) -> ()
                n4358 = local write "FIB"(w3256) -> ()
              }
            }
          }
          event "Pause for reheat": Value Change {
            n4359 = event-data() -> ("NewVal"=w3308:bool)  [unwired: 6 out]
            n4360 = case shown="False" w3308 {
              frame False {
                w3311 = u8 0 ("FI below limit counts")
                n4361 = local read "Machine Type"() -> (w3309:u8)
                n4362 = case shown="0, Default" w3309 {
                  tunnel: [w3317 w3325 w3326] -> w3310
                  frame 0, Default {
                    n4363 = for {
                      N: 10 -> [_]
                      tunnel: [w3322] -> w3319 mode=indexing
                      n4364 = shared-variable ".\\Zeiss Library.lvlib\\Logs"() -> (w3324:sgl[])  [unwired: 1 in, 1 out]
                      n4365 = Wait Until Next ms Multiple(millisecond multiple=u32 10) -> ()  [unwired: 1 out]
                      n4366 = Index Array(array=w3324, index=0) -> (element=w3322:sgl)
                    }
                    n4367 = call-poly <vilib>:"Basic Averaged DC-RMS.vi"("signal in"=w3319) -> ("DC value"=w3318:dbl)  [unwired: 7 in, 3 out]
                    n4368 = To Single Precision Float(number=w3318) -> (single precision float=w3317:sgl)
                  }
                  frame 1 {
                    n4369 = local read "Faraday Cup (nA)"() -> (w3325:sgl)
                  }
                  frame 2 {
                    n4370 = for {
                      N: 10 -> [_]
                      tunnel: [w3331] -> w3328 mode=indexing
                      n4371 = shared-variable ".\\Zeiss Library.lvlib\\Logs"() -> (w3333:sgl[])  [unwired: 1 in, 1 out]
                      n4372 = Wait Until Next ms Multiple(millisecond multiple=u32 10) -> ()  [unwired: 1 out]
                      n4373 = Index Array(array=w3333, index=0) -> (element=w3331:sgl)
                    }
                    n4374 = call-poly <vilib>:"Basic Averaged DC-RMS.vi"("signal in"=w3328) -> ("DC value"=w3327:dbl)  [unwired: 7 in, 3 out]
                    n4375 = To Single Precision Float(number=w3327) -> (single precision float=w3326:sgl)
                  }
                }
                n4376 = local write "FI below limit counts"(w3311) -> ()
                n4377 = local write "FIB CL I out of bound counts"(w3311) -> ()
                n4378 = shared-variable ".\\Zeiss Library.lvlib\\Faraday Cup before mill"(w3310) -> ()  [unwired: 1 in, 1 out]
